vi "Write friction.vi"(8 "error in (no error)":errorcluster, 10 "friction":dbl, 11 "GameObject in":refnum<class "GameObject.lvclass">) -> (0 "error out":errorcluster, 3 "GameObject out":refnum<class "GameObject.lvclass">)   [LabVIEW 2019, in "RT_Game.lvlib" / "GameObject.lvclass"]
uses:
  GameObject.lvclass
  GameObject.lvclass/GameObject.ctl
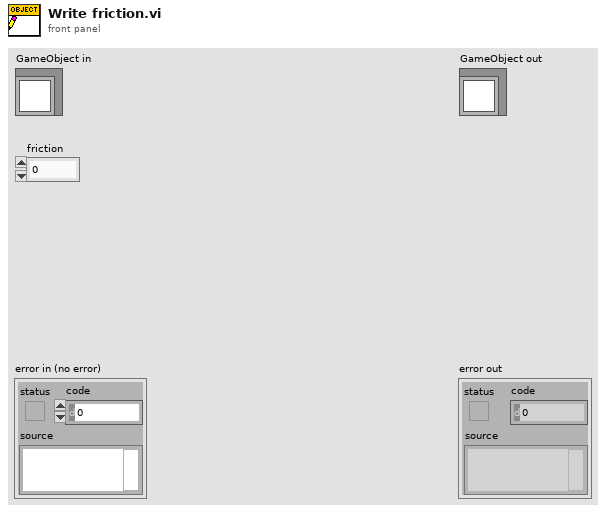
[diagram p1: front panel]
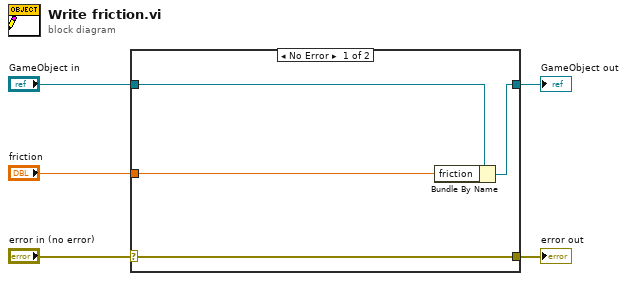
[diagram p0: block diagram]
diagram:
  n1 = case shown="No Error" "error in (no error)" {
    selector: "error in (no error)" -> [w9 w10]
    tunnel: [w9 w10] -> w4
    tunnel: [w7 w11] -> w2
    tunnel: "GameObject in" -> [w8 w11]
    tunnel: "friction" -> [w6 _]
    frame No Error {
      n2 = Bundle By Name(cluster=w8, "friction"=w6) -> (w7:refnum<class "GameObject.lvclass">)
    }
    frame Error {
    }
  }
  "error out" <- w4
  "GameObject out" <- w2
